vi "Square_Root.vi"() -> ()   [LabVIEW 2020]
panel:
  out "output variable":dbl
  in  "input variable":dbl
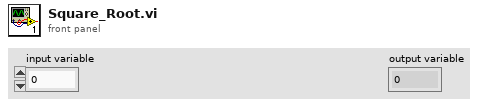
[diagram p1: front panel]
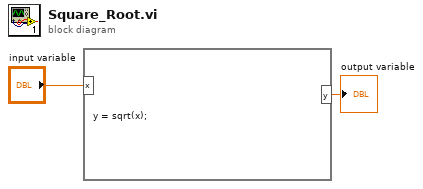
[diagram p0: block diagram]
diagram:
  n1 = formula code="y = sqrt(x);"("x"="input variable") -> ("y"=→"output variable":dbl)
